vi "Write HostName.vi"(8 "error in (no error)":errorcluster, 10 "HostName":string, 11 "CI Project in":refnum<class "CI Project.lvclass">) -> (0 "error out":errorcluster, 3 "CI Project out":refnum<class "CI Project.lvclass">)   [LabVIEW 2014, in "CI Project.lvclass"]
uses:
  CI Project.lvclass
  CI Project.lvclass/CI Project.ctl
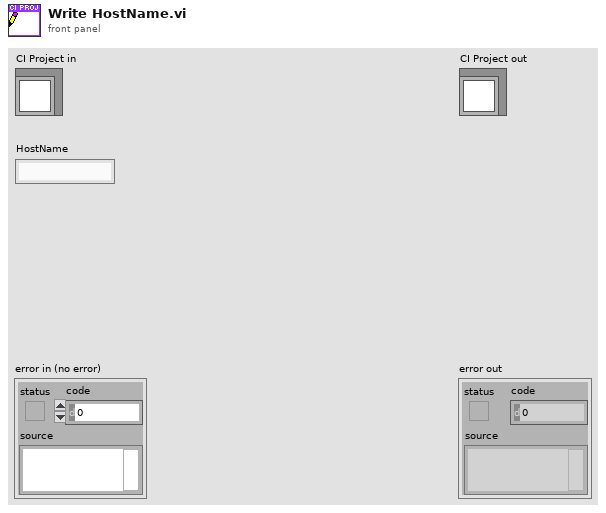
[diagram p1: front panel]
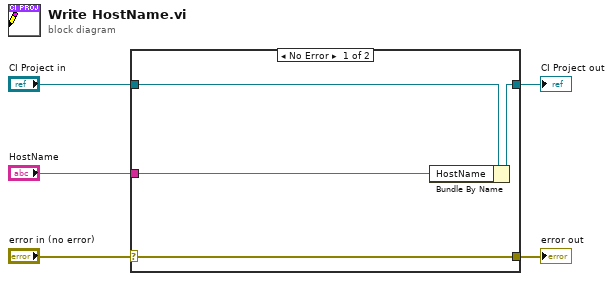
[diagram p0: block diagram]
diagram:
  n1 = case shown="No Error" "error in (no error)" {
    selector: "error in (no error)" -> [w9 w10]
    tunnel: [w9 w10] -> w4
    tunnel: [w7 w11] -> w2
    tunnel: "CI Project in" -> [w8 w11]
    tunnel: "HostName" -> [w6 _]
    frame No Error {
      n2 = Bundle By Name(cluster=w8, "HostName"=w6) -> (w7:refnum<class "CI Project.lvclass">)
    }
    frame Error {
    }
  }
  "error out" <- w4
  "CI Project out" <- w2
